vi "Finish.vi"   [LabVIEW 2025]
doc: "This VI is called just before exiting. It is expected to close I/O refnum, save collected data, etc."
uses:
  <vilib>/Rock Robotics/WPI/Utilities/WPI_GetSetVariantRefNum.vi
types:
  T1 = typedef "WPI_JoystickDevRef.ctl" = cluster{"Device":T2}
  T2 = typedef "WPI_JoystickDeviceEnum.ctl" = enum16{"USB 0", "USB 1", "USB 2", "USB 3", "USB 4", "USB 5"}
  T3 = typedef "WPI_MotorControlDeviceRef.ctl" = cluster{"DeviceStatus":errorcluster, "Type":T4, "PWM":cluster{"PWM Channel":T5, "DeadBand":T6}, "CAN":cluster{"Device Number":u8, "SetOutput VI Ref":variant, "GetOutput VI Ref":variant, "Enable VI Ref":variant, "Disable VI Ref":variant, "Data":variant}, "Invert":bool, "DIO PWM":cluster{"PWM \"Enable\" Channel":T5, "DIOChannel":T7, "PWM Rate":dbl}}
  T4 = typedef "WPI_MotorControlType.ctl" = enum16{"PWM", "CAN", "DIO PWM"}
  T5 = typedef "FPGA_DIOPWMChannel.ctl" = enum8{"PWM 0", "PWM 1", "PWM 2", "PWM 3", "PWM 4", "PWM 5", "PWM 6", "PWM 7", "PWM 8", "PWM 9", "PWM MXP 0", "PWM MXP 1", "PWM MXP 2", "PWM MXP 3", "PWM MXP 4", "PWM MXP 5", "PWM MXP 6", "PWM MXP 7", "PWM MXP 8", "PWM MXP 9", "Invalid"}
  T6 = typedef "WPI_PWMDeadband.ctl" = cluster{"Name":string, "maxPositivePwm":i32, "minPositivePwm":i32, "centerPwm":i32, "maxNegativePwm":i32, "minNegativePwm":i32, "angularRange":u16}
  T7 = typedef "FPGA_DIOChannel.ctl" = enum8{"DIO 0", "DIO 1", "DIO 2", "DIO 3", "DIO 4", "DIO 5", "DIO 6", "DIO 7", "DIO 8", "DIO 9", "DIO MXP 0", "DIO MXP 1", "DIO MXP 2", "DIO MXP 3", "DIO MXP 4", "DIO MXP 5", "DIO MXP 6", "DIO MXP 7", "DIO MXP 8", "DIO MXP 9", "DIO MXP 10", "DIO MXP 11", "DIO MXP 12", "DIO MXP 13", "DIO MXP 14", "DIO MXP 15", "SPI Port CS1", "SPI Port CS2", "SPI Port CS3", "SPI Port MISO", "SPI Port MOSI", "Invalid"}
  T8 = typedef "WPI_ServoDeviceRef.ctl" = cluster{"DeviceStatus":errorcluster, "PWM Channel":T5, "DeadBand":T6}
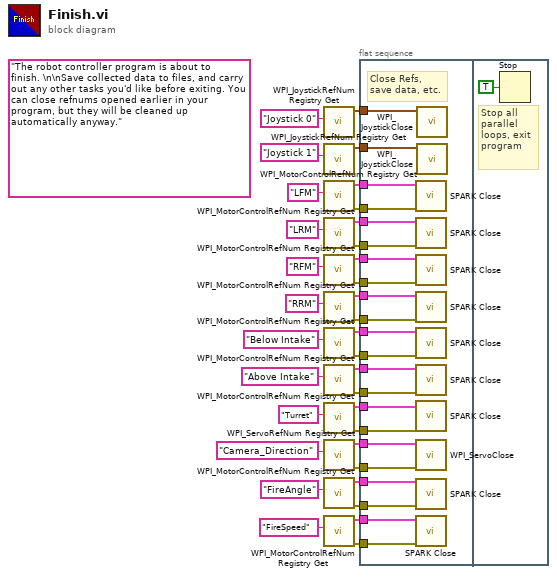
[diagram p0: block diagram]
diagram:
  (unwired) "The robot controller program is about to finish. \n\nSave collected data to files, and carry out any other tasks you'd like before exiting. You can close refnums opened earlier in your program, but they will be cleaned up automatically anyway."
  n1 = call <vilib>:"WPI_JoystickRefNum Registry Get.vi"("refnum name"="Joystick 0") -> ("JoystickDevRef"=w33:T1)  [unwired: 1 in, 9 out]
  n2 = call <vilib>:"WPI_JoystickRefNum Registry Get.vi"("refnum name"="Joystick 1") -> ("JoystickDevRef"=w10:T1)  [unwired: 1 in, 9 out]
  n3 = call <vilib>:"WPI_MotorControlRefNum Registry Get.vi"("refnum name"="LFM") -> ("error out"=w28:errorcluster, "MotorControlDevRef"=w27:T3)  [unwired: 9 in]
  n4 = call <vilib>:"WPI_MotorControlRefNum Registry Get.vi"("refnum name"="LRM") -> ("error out"=w22:errorcluster, "MotorControlDevRef"=w21:T3)  [unwired: 9 in]
  n5 = call <vilib>:"WPI_MotorControlRefNum Registry Get.vi"("refnum name"="RFM") -> ("error out"=w24:errorcluster, "MotorControlDevRef"=w23:T3)  [unwired: 9 in]
  n6 = call <vilib>:"WPI_MotorControlRefNum Registry Get.vi"("refnum name"="RRM") -> ("error out"=w26:errorcluster, "MotorControlDevRef"=w25:T3)  [unwired: 9 in]
  n7 = call <vilib>:"WPI_MotorControlRefNum Registry Get.vi"("refnum name"="Below Intake") -> ("error out"=w16:errorcluster, "MotorControlDevRef"=w15:T3)  [unwired: 9 in]
  n8 = call <vilib>:"WPI_MotorControlRefNum Registry Get.vi"("refnum name"="Above Intake") -> ("error out"=w18:errorcluster, "MotorControlDevRef"=w17:T3)  [unwired: 9 in]
  n9 = call <vilib>:"WPI_MotorControlRefNum Registry Get.vi"("refnum name"="Turret") -> ("error out"=w7:errorcluster, "MotorControlDevRef"=w8:T3)  [unwired: 9 in]
  n10 = call <vilib>:"WPI_ServoRefNum Registry Get.vi"("refnum name"="Camera_Direction") -> ("error out"=w13:errorcluster, "ServoDeviceRef"=w14:T8)  [unwired: 9 in]
  n11 = call <vilib>:"WPI_MotorControlRefNum Registry Get.vi"("refnum name"="FireAngle") -> ("error out"=w5:errorcluster, "MotorControlDevRef"=w4:T3)  [unwired: 9 in]
  n12 = call <vilib>:"WPI_MotorControlRefNum Registry Get.vi"("refnum name"="FireSpeed") -> ("error out"=w2:errorcluster, "MotorControlDevRef"=w1:T3)  [unwired: 9 in]
  n13 = flat-sequence {
    tunnel: w33 -> [w56]
    tunnel: w28 -> [w55]
    tunnel: w27 -> [w54]
    tunnel: w26 -> [w53]
    tunnel: w25 -> [w52]
    tunnel: w24 -> [w51]
    tunnel: w23 -> [w50]
    tunnel: w22 -> [w49]
    tunnel: w21 -> [w48]
    tunnel: w18 -> [w47]
    tunnel: w17 -> [w46]
    tunnel: w16 -> [w45]
    tunnel: w15 -> [w44]
    tunnel: w14 -> [w43]
    tunnel: w13 -> [w42]
    tunnel: w10 -> [w41]
    tunnel: w8 -> [w40]
    tunnel: w7 -> [w39]
    tunnel: w5 -> [w38]
    tunnel: w4 -> [w37]
    tunnel: w2 -> [w36]
    tunnel: w1 -> [w35]
    frame #0 {
      # "Close Refs, save data, etc."
      n14 = call <vilib>:"SPARK Close.vi"("error in"=w55, "MotorControlDeviceRef"=w54) -> ()  [unwired: 9 in, 1 out]
      n15 = call <vilib>:"SPARK Close.vi"("error in"=w49, "MotorControlDeviceRef"=w48) -> ()  [unwired: 9 in, 1 out]
      n16 = call <vilib>:"SPARK Close.vi"("error in"=w51, "MotorControlDeviceRef"=w50) -> ()  [unwired: 9 in, 1 out]
      n17 = call <vilib>:"SPARK Close.vi"("error in"=w53, "MotorControlDeviceRef"=w52) -> ()  [unwired: 9 in, 1 out]
      n18 = call <vilib>:"SPARK Close.vi"("error in"=w45, "MotorControlDeviceRef"=w44) -> ()  [unwired: 9 in, 1 out]
      n19 = call <vilib>:"SPARK Close.vi"("error in"=w47, "MotorControlDeviceRef"=w46) -> ()  [unwired: 9 in, 1 out]
      n20 = call <vilib>:"SPARK Close.vi"("error in"=w39, "MotorControlDeviceRef"=w40) -> ()  [unwired: 9 in, 1 out]
      n21 = call <vilib>:"WPI_ServoClose.vi"("error in (no error)"=w42, "ServoDeviceRef"=w43) -> ()  [unwired: 9 in, 1 out]
      n22 = call <vilib>:"SPARK Close.vi"("error in"=w38, "MotorControlDeviceRef"=w37) -> ()  [unwired: 9 in, 1 out]
      n23 = call <vilib>:"SPARK Close.vi"("error in"=w36, "MotorControlDeviceRef"=w35) -> ()  [unwired: 9 in, 1 out]
      n24 = call <vilib>:"WPI_JoystickClose.vi"("JoystickDevRef"=w56) -> ()  [unwired: 11 out]
      n25 = call <vilib>:"WPI_JoystickClose.vi"("JoystickDevRef"=w41) -> ()  [unwired: 11 out]
    }
    frame #1 {
      # "Stop all parallel\nloops, exit program"
      n26 = Stop(stop? (T)=TRUE ("Quit")) -> ()
    }
  }
